vi "AssetMgrQueryAssetNodeViewsResponse_Parse.vi"(8 "error in (no error)":errorcluster, 11 "Message":T9) -> (0 "error out":errorcluster, 1 "Body":T1, 2 "Header":T8, 3 "AssetMgrQueryAssetNodeViewsResponse":T7)   [LabVIEW 2017]
uses:
  <vilib>/addons/InsightCM/MessageBus/Base/controls/Message.ctl
  <vilib>/addons/InsightCM/MessageBus/Base/controls/MessageHeader.ctl
  <vilib>/addons/InsightCM/MessageBus/Base/controls/KeyValuePair.ctl
  <vilib>/addons/InsightCM/MessageBus/MessageLibrary/AssetManager/controls/AssetMgrQueryAssetNodeViewsResponse.ctl
  <vilib>/addons/InsightCM/MessageBus/MessageLibrary/AssetManager/controls/AssetMgrQueryAssetNodeViewsResponseBody.ctl
  <vilib>/addons/InsightCM/MessageBus/Base/controls/AssetNodeView.ctl
  <vilib>/addons/InsightCM/MessageBus/Base/controls/AssetState.ctl
  <vilib>/addons/InsightCM/MessageBus/Base/controls/Metric.ctl
  <vilib>/addons/InsightCM/MessageBus/Base/controls/AssetNodeReference.ctl
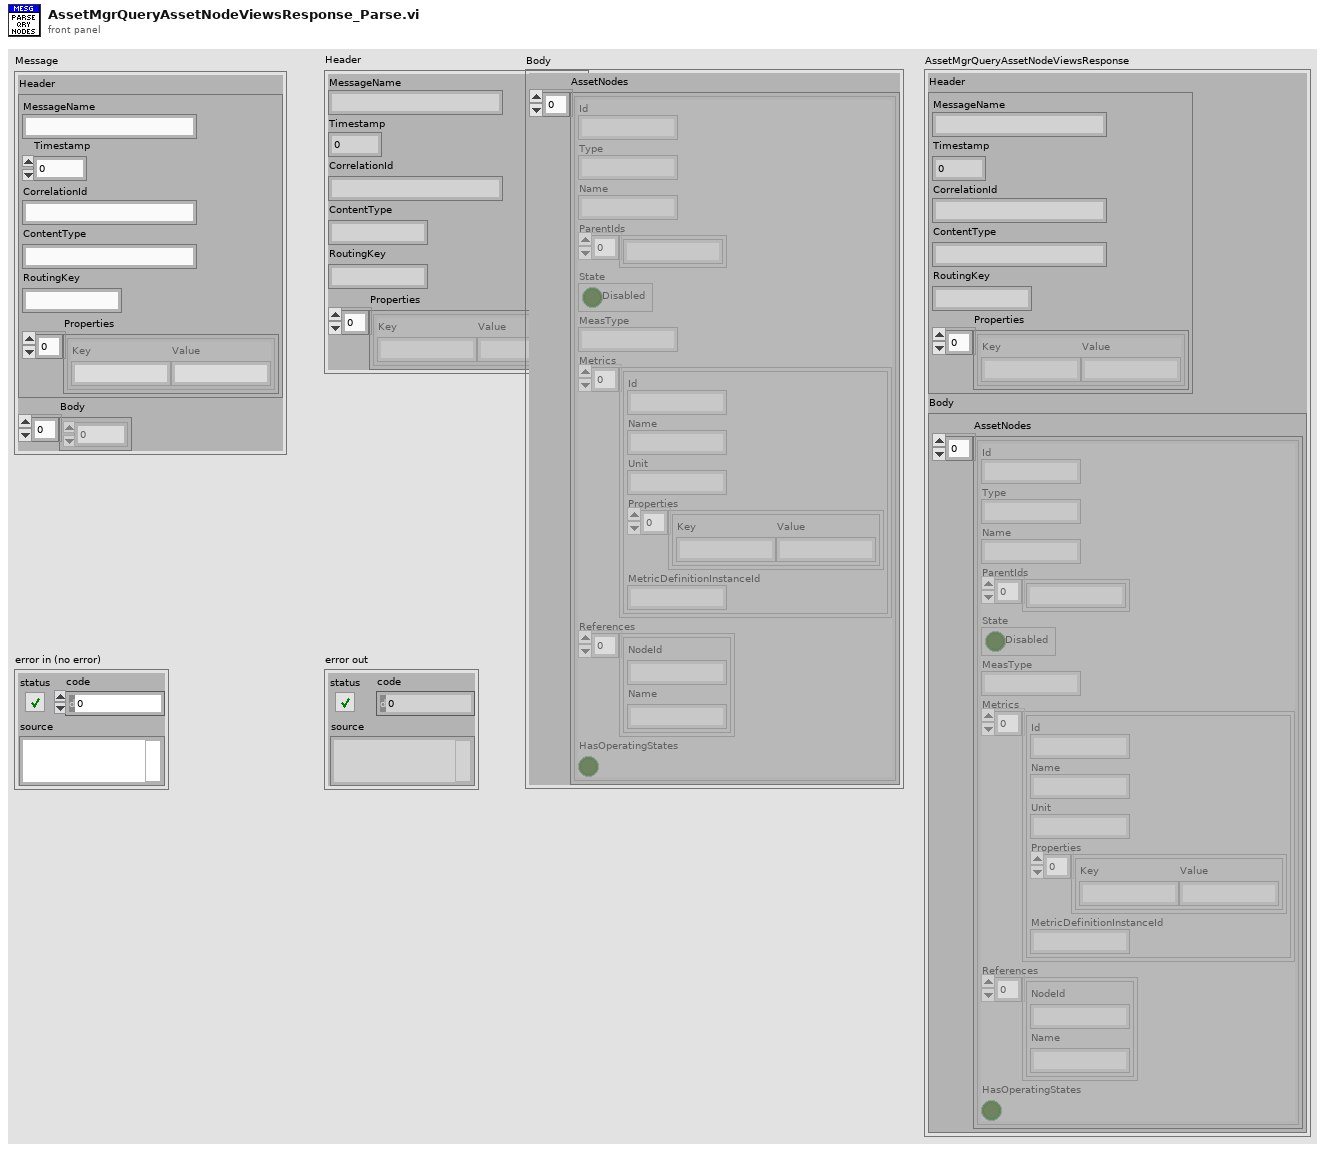
[diagram p1: front panel]
types:
  T1 = typedef "AssetMgrQueryAssetNodeViewsResponseBody.ctl" = cluster{"AssetNodes":T2[]}
  T2 = typedef "AssetNodeView.ctl" = cluster{"Id":string, "Type":string, "Name":string, "ParentIds":string[], "State":T3, "MeasType":string, "Metrics":T4[], "References":T6[], "HasOperatingStates":bool}
  T3 = typedef "AssetState.ctl" = cluster{"Disabled":bool}
  T4 = typedef "Metric.ctl" = cluster{"Id":string, "Name":string, "Unit":string, "Properties":T5[], "MetricDefinitionInstanceId":string}
  T5 = typedef "KeyValuePair.ctl" = cluster{"Key":string, "Value":string}
  T6 = typedef "AssetNodeReference.ctl" = cluster{"NodeId":string, "Name":string}
  T7 = typedef "AssetMgrQueryAssetNodeViewsResponse.ctl" = cluster{"Header":T8, "Body":T1}
  T8 = typedef "MessageHeader.ctl" = cluster{"MessageName":string, "Timestamp":i64, "CorrelationId":string, "ContentType":string, "RoutingKey":string, "Properties":T5[]}
  T9 = typedef "Message.ctl" = cluster{"Header":T8, "Body":u8[]}
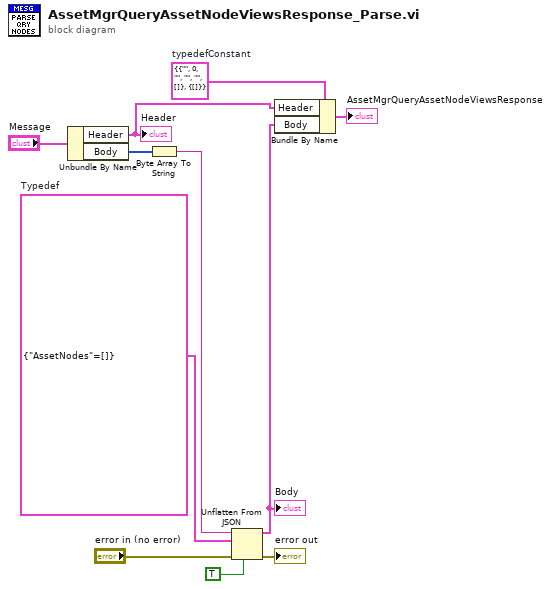
[diagram p0: block diagram]
diagram:
  w3 = T7 {"Header"={"MessageName"="", "Timestamp"=0, "CorrelationId"="", "ContentType"="", "RoutingKey"="", "Properties"=[]}, "Body"={"AssetNodes"=[]}}  # typedefConstant
  w7 = T1 {"AssetNodes"=[]}  # Typedef
  n1 = Unbundle By Name("Message") -> ("Header"=w9:T8, "Body"=w1:u8[])
  "Header" <- w9
  n2 = Byte Array To String(unsigned byte array=w1) -> (string=w6:string)
  n3 = Unflatten From JSON(JSON string=w6, type and defaults=w7, default null elements? (F)=TRUE, error in (no error)="error in (no error)") -> (value=w5:T1, error out=→"error out":errorcluster)  [unwired: 3 in]
  "Body" <- w5
  n4 = Bundle By Name(cluster=w3, "Header"=w9, "Body"=w5) -> (→"AssetMgrQueryAssetNodeViewsResponse":T7)
